vi "Global.vi"() -> ()   [LabVIEW 2013]
uses:
  <userlib>/KNR OS 3.0 LabVIEW Toolkit/Type Definition/DC Motor Port.ctl
panel:
  out "Control_definition":T1
  out "KNR_definition":T3={"MM2DEG"=0.0, "PLS2DEG"=0.0, "Ts"=0.0, "Tcnt"=0, "fs"=0, "Vmax"=0.0, "Jmax"=0.0, "N_Delay"=0, "C_port"=4, "KNRPLS"=0.0} {"C_port" items=["DS1"=4, "DS2"=5, "DS3"=6, "DS4"=7]}
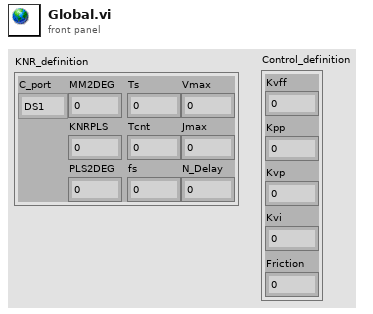
[diagram p1: front panel]
types:
  T1 = cluster{"Kvff":dbl, "Kpp":dbl, "Kvp":dbl, "Kvi":dbl, "Friction":dbl}
  T2 = typedef "DC Motor Port.ctl" = u16
  T3 = cluster{"MM2DEG":dbl, "PLS2DEG":dbl, "Ts":dbl, "Tcnt":i32, "fs":i32, "Vmax":dbl, "Jmax":dbl, "N_Delay":i32, "C_port":T2, "KNRPLS":dbl}
diagram:
